vi "testcase - INI-Static-Variable-Support.vi"() -> ()   [LabVIEW 2017]
uses:
  <userlib>/_NEVSTOP/Communicable State Machine(CSM)/Communicable State Machine.lvlib
  INI-Static-Variable-Support/INI-Static-Variable-Support.lvlib
panel:
  in  "String 2":string="Data: Load Configuration >> ip:${ip:127.0.0.1};port:${port:5000} -> NetworkModule\nData: Load Configuration >> ${ip:127.0.0.1}:${port:5000} -> NetworkModule\nData: Load Configuration >> ip:${ip} -> NetworkModule\nData: Load Configuration >> ${port:5000} -> NetworkModule"
  out "String":string="Data: Load Configuration >> ip:https:%2F%2Fwww.ni.com;port:443 -> NetworkModule\r\nData: Load Configuration >> https:%2F%2Fwww.ni.com:443 -> NetworkModule\r\nData: Load Configuration >> ip:https:%2F%2Fwww.ni.com -> NetworkModule\r\nData: Load Configuration >> 443 -> NetworkModule"
  out "error out":errorcluster
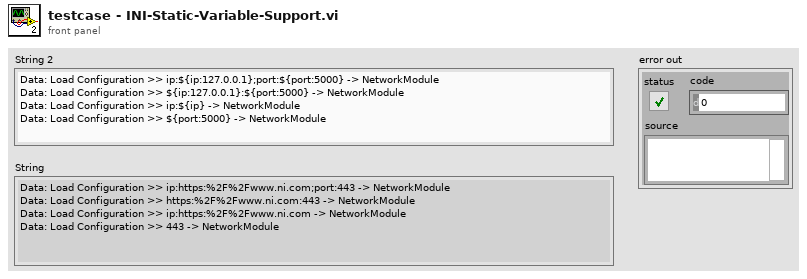
[diagram p1: front panel]
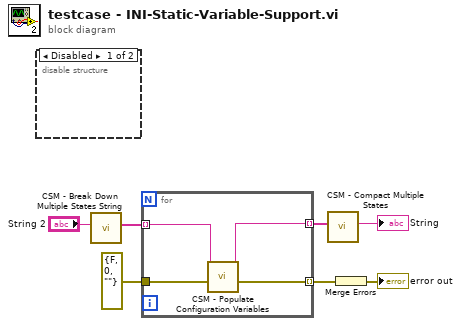
[diagram p0: block diagram]
diagram:
  n1 = disable-structure shown="Disabled" {
    frame Disabled {
    }
    frame Enabled {
    }
  }
  n2 = call <userlib>:"CSM - Break Down Multiple States String.vi"("States"="String 2") -> ("Multiple States"=w2:string[])  [unwired: 10 in]
  n3 = for {
    tunnel: [w11] -> w6 mode=indexing
    tunnel: w2 -> [w10] mode=indexing
    tunnel: errorcluster {"status"=FALSE, "code"=0, "source"=""} ("error out") -> [w9]
    tunnel: [w8] -> w7 mode=indexing
    n4 = call "CSM - Populate Configuration Variables.vi"("error in (no error)"=w9, "String in"=w10) -> ("error out"=w8:errorcluster, "String out"=w11:string)  [unwired: 6 in]
  }
  n5 = call <userlib>:"CSM - Compact Multiple States.vi"("Multiple States"=w6) -> ("States"=→"String":string)  [unwired: 9 in]
  n6 = Merge Errors(w7) -> (→"error out":errorcluster)
